vi "Write States.vi"(8 "error in (no error)":errorcluster, 10 "States":T1=enum."KickToGoal", 11 "ShootTactic in":refnum<class "ShootTactic.lvclass">) -> (0 "error out":errorcluster, 3 "ShootTactic out":refnum<class "ShootTactic.lvclass">)   [LabVIEW 2023, in "ShootTactic.lvclass"]
uses:
  ShootTactic.lvclass
  States.ctl
  ShootTactic.lvclass/ShootTactic.ctl
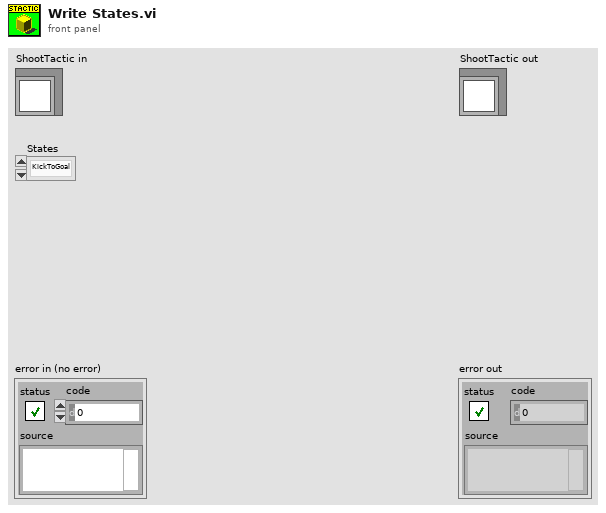
[diagram p1: front panel]
types:
  T1 = typedef "ShootTactic.lvclass/States.ctl" = enum16{"BallInGoalieArea", "Exit", "KickToGoal", "InterceptBall"}
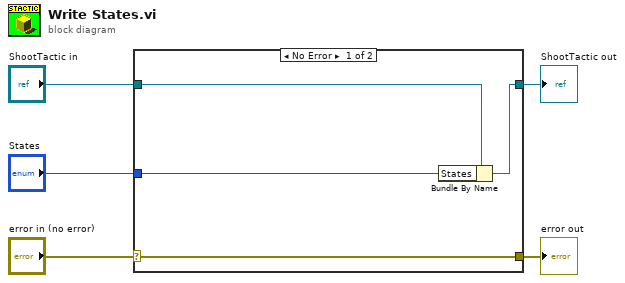
[diagram p0: block diagram]
diagram:
  n1 = case shown="No Error" "error in (no error)" {
    selector: "error in (no error)" -> [w9 w10]
    tunnel: [w9 w10] -> w4
    tunnel: [w7 w11] -> w2
    tunnel: "ShootTactic in" -> [w8 w11]
    tunnel: "States" -> [w6 _]
    frame No Error {
      n2 = Bundle By Name(cluster=w8, "States"=w6) -> (w7:refnum<class "ShootTactic.lvclass">)
    }
    frame Error {
    }
  }
  "error out" <- w4
  "ShootTactic out" <- w2
